vi "Sum Big Integer.vi"(10 "y":string, 11 "x":string) -> (3 "x+y":string)   [LabVIEW 2013, in "Problem 16.lvlib"]
uses:
  Problem 16.lvlib
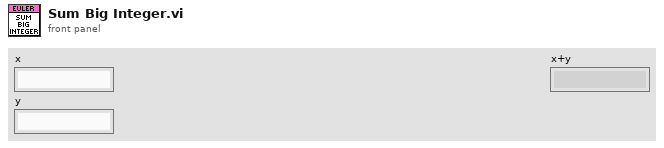
[diagram p1: front panel]
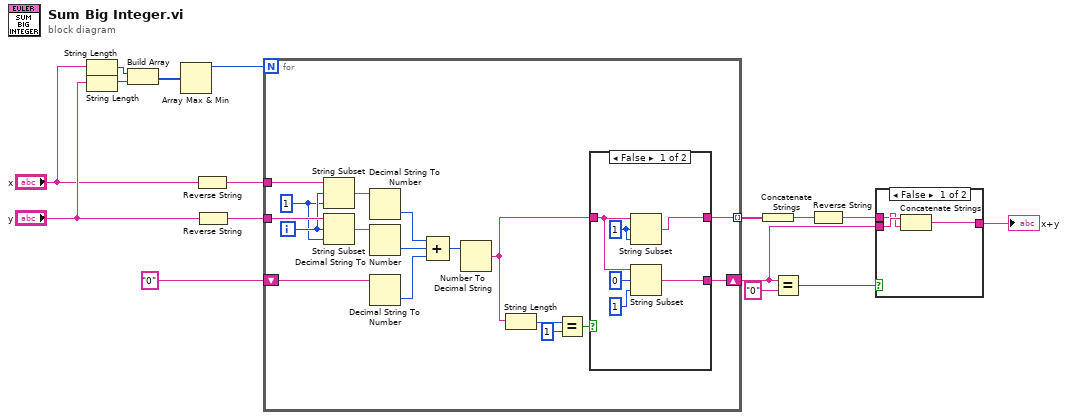
[diagram p0: block diagram]
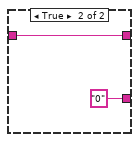
[diagram p3: hidden frame]
diagram:
  n1 = String Length(string="x") -> (length=w5:i32)
  n2 = String Length(string="y") -> (length=w4:i32)
  n3 = Build Array(w5, w4) -> (w3:i32[])
  n4 = Array Max & Min(array=w3) -> (max value=w2:i32)  [unwired: 3 out]
  n5 = Reverse String(1:"x") -> (0:w15:string)
  n6 = Reverse String(1:"y") -> (0:w14:string)
  n7 = for {
    N: w2 -> [_]
    tunnel: w15 -> [w33]
    tunnel: w14 -> [w32]
    shift-right: [w17] -> w9
    shift-left: "0" -> [w27]
    tunnel: [w19] -> w13 mode=indexing
    i -> [w31]
    w30 = 1 ("length (rest)")
    n8 = String Subset(string=w33, offset (0)=w31, length (rest)=w30) -> (substring=w29:string)
    n9 = String Subset(string=w32, offset (0)=w31, length (rest)=w30) -> (substring=w28:string)
    n10 = Decimal String To Number(string=w29) -> (number=w26:i32)  [unwired: 2 in, 1 out]
    n11 = Decimal String To Number(string=w28) -> (number=w24:i32)  [unwired: 2 in, 1 out]
    n12 = Decimal String To Number(string=w27) -> (number=w25:i32)  [unwired: 2 in, 1 out]
    n13 = Compound Arithmetic op=ADD(w26, w24, w25) -> (w23:i32)
    n14 = Number To Decimal String(number=w23) -> (decimal integer string=w20:string)  [unwired: 1 in]
    n15 = String Length(string=w20) -> (length=w22:i32)
    n16 = Equal?(x=w22, y=1) -> (x = y?=w18:bool)
    n17 = case shown="False" w18 {
      tunnel: w20 -> [w36 w41]
      tunnel: [w34 w41] -> w19
      tunnel: [w37 "0"] -> w17
      frame False {
        w35 = 1 ("offset (0)")
        n18 = String Subset(string=w36, offset (0)=w35, length (rest)=w35) -> (substring=w34:string)
        n19 = String Subset(string=w36, offset (0)=0, length (rest)=1 ("length (rest)")) -> (substring=w37:string)
      }
      frame True {
      }
    }
  }
  n20 = Concatenate Strings(w13) -> (w10:string)
  n21 = Equal?(x=w9, y="0") -> (x = y?=w11:bool)
  n22 = Reverse String(1:w10) -> (0:w1:string)
  n23 = case shown="False" w11 {
    tunnel: w1 -> [w42 w45]
    tunnel: w9 -> [w43 _]
    tunnel: [w44 w45] -> w8
    frame False {
      n24 = Concatenate Strings(w43, w42) -> (w44:string)
    }
    frame True {
    }
  }
  "x+y" <- w8
